vi "SetLogPath.vi"(8 "error in (no error)":errorcluster, 10 "LogPath":path) -> (0 "error out":errorcluster)   [LabVIEW 2014, in "GCMLog.lvclass"]
uses:
  GCMLog.lvclass
  GCMLogGlobals.vi
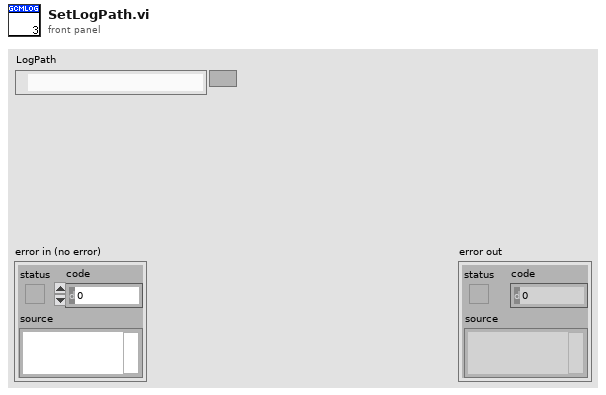
[diagram p1: front panel]
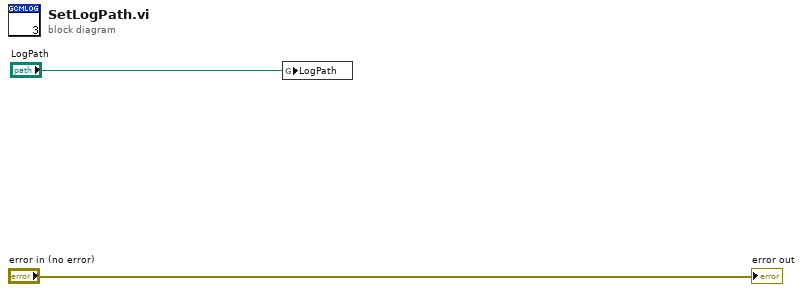
[diagram p0: block diagram]
diagram:
  n1 = global write "GCMLogGlobals.vi" "LogPath"("LogPath") -> ()
  "error out" <- "error in (no error)"
